vi "Main.vi"(11 "Module Admin":refnum<class "Delacor_lib_QMH_Module Admin.lvclass">) -> ()   [LabVIEW 2021, in "Hardware Selection.lvlib"]
doc: "This template is based off of the Queued Message Handler design pattern and the Queued Message Handler project template that ships with LabVIEW.\n\nThe main difference is that the queue is private to this module and communication between modules is performed via Broadcast and Request events.\n\nRequest events are wrapped in public API methods and are handled in the Event Handling Loop (EHL) of this VI. Any module can register for Broadcast events sent by this module. The EHL generates messages based on user interface actions.\n\nThe Message Handling Loop (MHL) processes messages generated by the EHL, or by other messages. The messages are string values, so new messages can be added easily to the Message Cases case structure in the MHL. Each message cluster can also provide an optional value for Message Data, which is a variant that can be converted to whatever message-specific data is required.\n_____\nBased on DQMH Project Template 7.0.1.1316."
uses:
  Hardware Selection.lvlib
  <vilib>/Delacor/Delacor QMH/Libraries/Module Admin_class/Delacor_lib_QMH_Module Admin.lvclass
  Module Data--cluster.ctl
  <vilib>/Delacor/Delacor QMH/Libraries/Message Queue_class/Delacor_lib_QMH_Message Queue.lvclass/Delacor_lib_QMH_Message Queue.ctl
  Stop Argument--cluster.ctl
  <vilib>/Delacor/Delacor QMH/Libraries/Module Admin_class/Delacor_lib_QMH_Module Admin.lvclass/Delacor_lib_QMH_Module Admin.ctl
  Get Selected RT Hardware Argument--cluster.ctl
  <vilib>/Utility/miscctls.llb/LVPointTypeDef.ctl
  Host-Control's/Module ID Action Enum.ctl
  Host-Control's/RT Exec FGV Action.ctl
  Host-Control's/DTT File's Name.ctl
  <vilib>/Delacor/Delacor QMH/Libraries/Message Queue_class/Delacor_lib_QMH_Enqueue Message (Single).vi
  <vilib>/Delacor/Delacor QMH/Libraries/Module Admin_class/Delacor_lib_QMH_Get External Launch.vi
  <userlib>/_OpenG.lib/array/array.llb/Search 1D Array (Boolean)__ogtk.vi
  <userlib>/_OpenG.lib/array/array.llb/Index 1D Array Elements (String)__ogtk.vi
  <vilib>/Delacor/Delacor QMH/Libraries/Message Queue_class/Delacor_lib_QMH_Message Queue.lvclass
  <userlib>/_OpenG.lib/array/array.llb/openg_array.lvlib
  <userlib>/_OpenG.lib/appcontrol/appcontrol.llb/openg_application_control.lvlib
panel:
  in  "DAQ-HW Selection":cluster{"Safety":bool, "Release":bool}
  in  "cDAQ-HW Data":cluster{"Hw Name":string, "Hw Ip":string}[](array[cluster])
  in  "RT-HW Selection":T1
  in  "RT-HW Data":cluster{"Hw Name":string, "Hw Ip":string}[](array[cluster])
  in  "Next":bool
  in  "Save IP":bool
  in  "Edit Tool":bool
  out "error out":errorcluster
  out "Status":string
  in  "Simulate MHL Error":bool
  in  "Simulate EHL Error":bool
  # "Hardware"
  # "IP-Address"
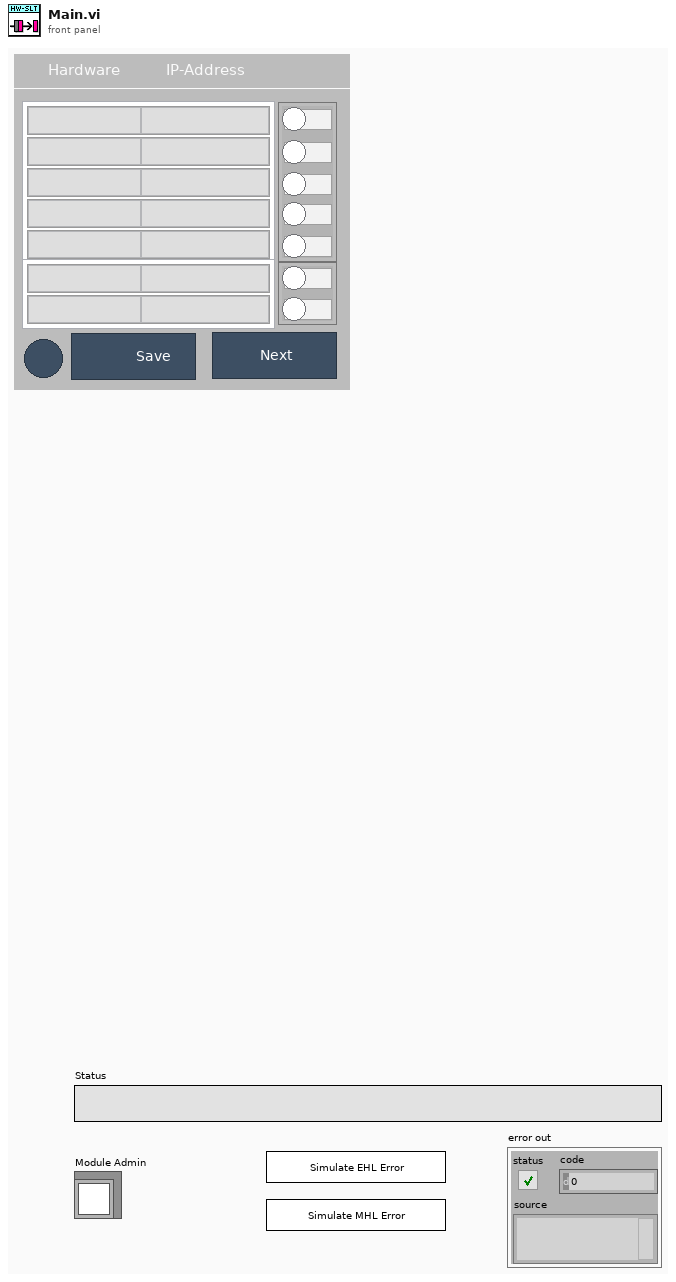
[diagram p1: front panel]
types:
  T1 = cluster{"Capsule-1":bool, "Capsule-2":bool, "Capsule-3":bool, "Capsule-4":bool, "sb-RIO":bool}
  T2 = typedef "Hardware Selection.lvlib/Request Events--cluster.ctl" = cluster{"Stop Module":refnum<user-event>, "Show Panel":refnum<user-event>, "Hide Panel":refnum<user-event>, "Get Module Execution Status":refnum<user-event>, "Show Diagram":refnum<user-event>, "Get Selected RT Hardware":refnum<user-event>}
  T3 = typedef "Hardware Selection.lvlib/Module Data--cluster.ctl" = cluster{"Status":string, "GUI Ref":cluster{"Hardware's":refnum<vi>, "IP Address":refnum<vi>}, "IP File Path":path, "HW Selection":cluster{"RT-HW Selection":cluster{"Capsule-1":bool, "Capsule-2":bool, "Capsule-3":bool, "Capsule-4":bool, "sb-RIO":bool}, "C-DAQ Hw Selection":cluster{"Safety":bool, "Release":bool}}, "IP File Data":cluster{"RT-Hw Name":string[], "cDAQ-Hw Name":string[], "RT-HW Enable?":bool[], "cDAQ-HW Enable?":bool[], "RT-HW IP":string[], "cDAQ-HW IP":string[]}, "Selected HW":cluster{"Slctd RT-Hw Name":string[], "Slctd RT-HW IP":string[], "Slctd cDAQ-Hw Name":string[], "Slctd cDAQ-HW IP":string[]}}
  T4 = cluster{"Ctrl.Label":string, "Ctrl.New Val":bool}
  T5 = enum32{"invalid lock state", "Not Locked", "Locked (No Password)", "Password-protected"}
  T6 = typedef "Hardware Selection.lvlib/Stop Argument--cluster.ctl" = cluster{"Origin":string, "Exit via Stop Module Req?":bool, "Wait for Module to stop?":bool}
  T7 = typedef "Hardware Selection.lvlib/Get Selected RT Hardware Argument--cluster.ctl" = cluster{"Get Slctd HW":bool}
  T8 = typedef "LVPointTypeDef.ctl" = cluster{"Horizontal":i16, "Vertical":i16}
  T9 = enum32{"Invalid", "Standard", "Closed", "Hidden", "Minimized", "Maximized"}
  T10 = typedef "RT Exec FGV Action.ctl" = enum16{"Init", "Insert", "Get a Exec?", "Get All Exec?"}
  T11 = typedef "Module ID Action Enum.ctl" = enum16{"Init", "Insert", "Get a ID", "Get all ID"}
  T12 = typedef "DTT File's Name.ctl" = enum16{"IP Address"}
  T13 = cluster{"RT-HW Enable?[0]":bool, "RT-HW Enable?[1]":bool, "RT-HW Enable?[2]":bool, "RT-HW Enable?[3]":bool, "RT-HW Enable?[4]":bool}
  T14 = cluster{"cDAQ-HW Enable?[0]":bool, "cDAQ-HW Enable?[1]":bool}
  T15 = cluster{"RT-Hw Name":string[], "cDAQ-Hw Name":string[], "RT-HW Enable?":bool[], "cDAQ-HW Enable?":bool[], "RT-HW IP":string[], "cDAQ-HW IP":string[]}
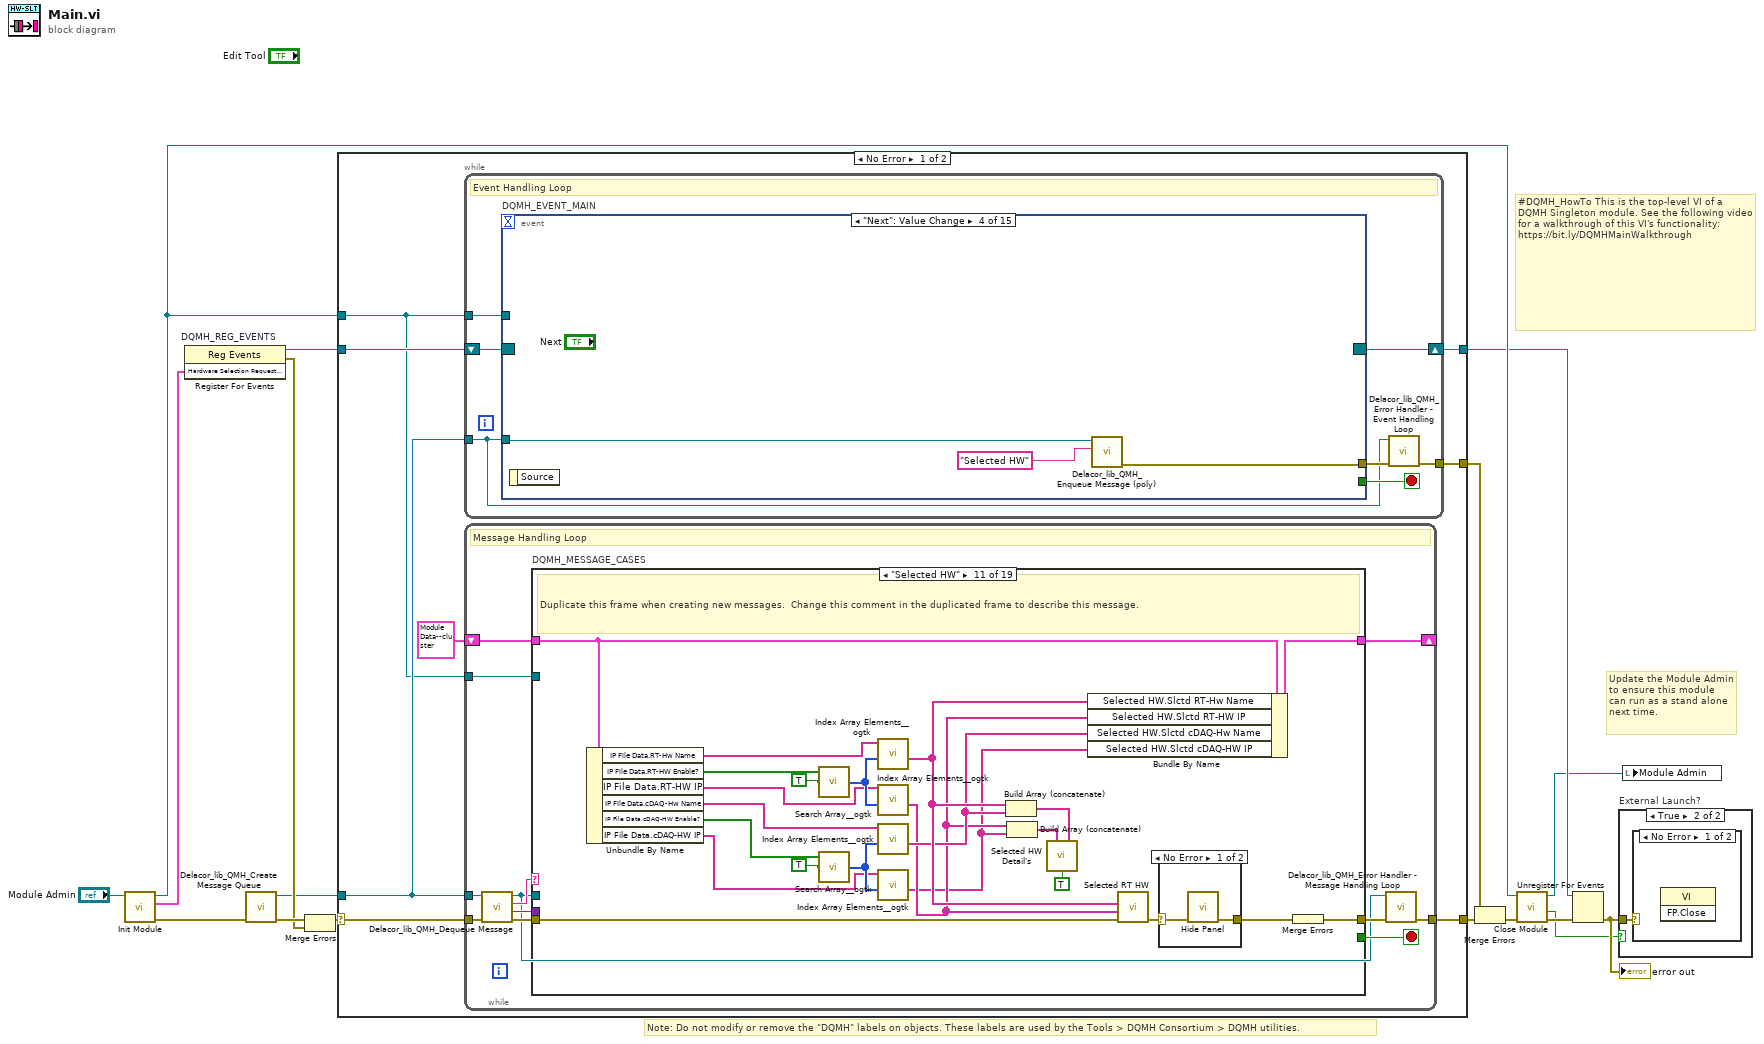
[diagram p0: block diagram]
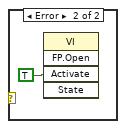
[diagram p3: hidden frame]
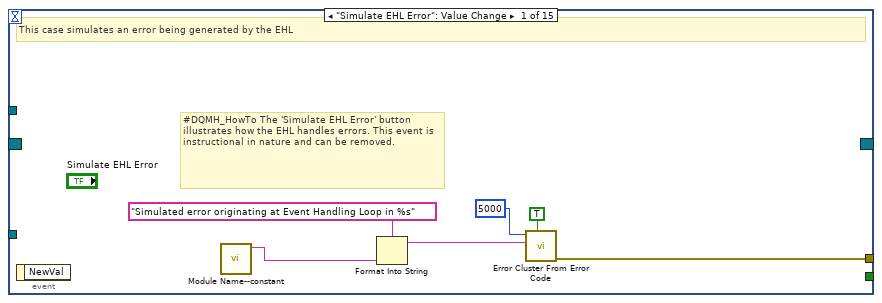
[diagram p4: hidden frame]
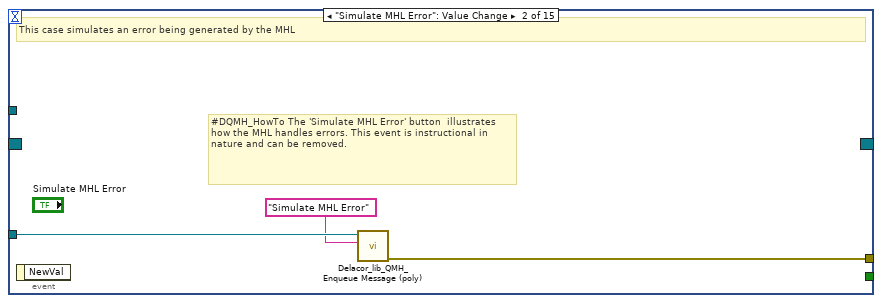
[diagram p5: hidden frame]
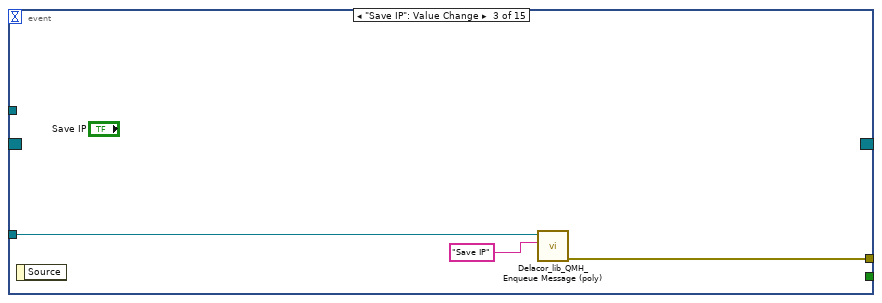
[diagram p6: hidden frame]
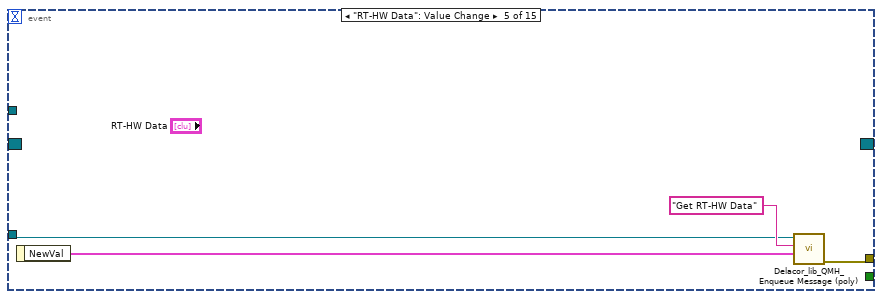
[diagram p7: hidden frame]
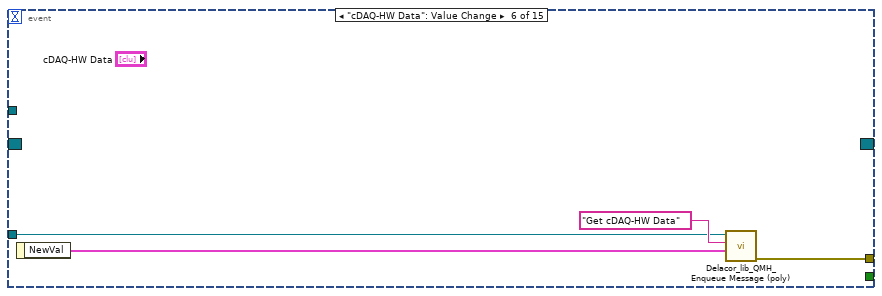
[diagram p8: hidden frame]
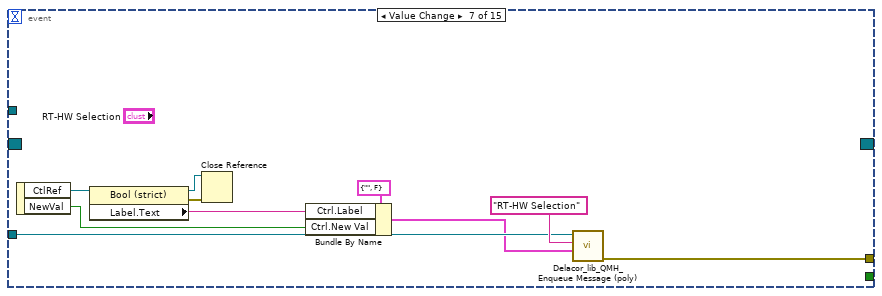
[diagram p9: hidden frame]
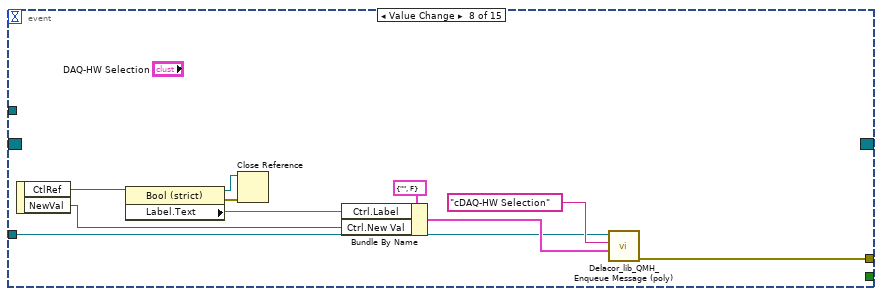
[diagram p10: hidden frame]
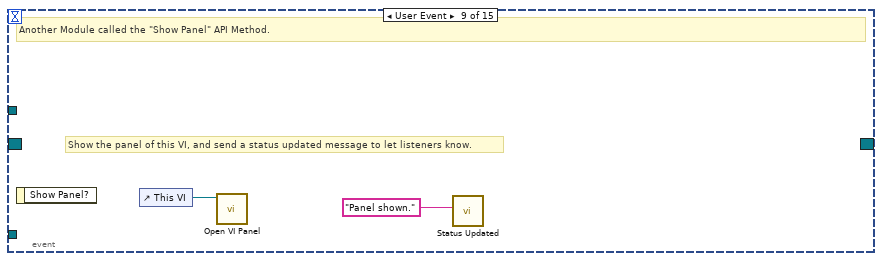
[diagram p11: hidden frame]
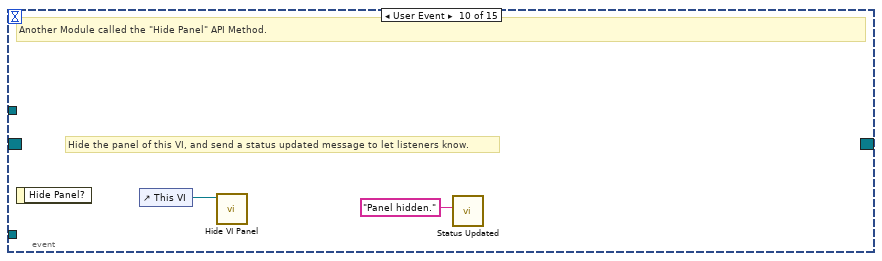
[diagram p12: hidden frame]
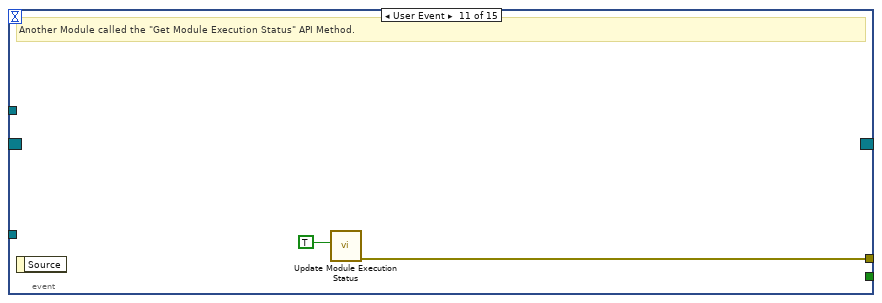
[diagram p13: hidden frame]
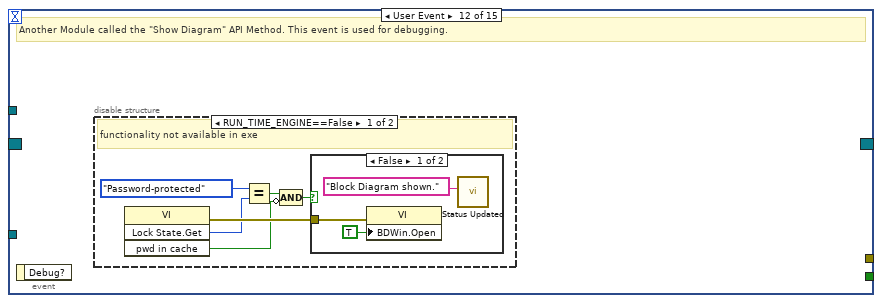
[diagram p14: hidden frame]
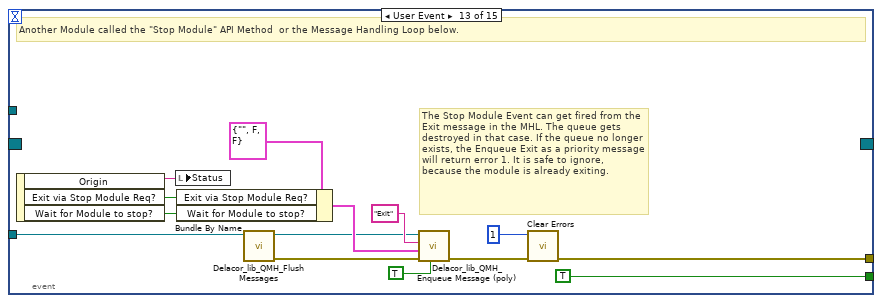
[diagram p17: hidden frame]
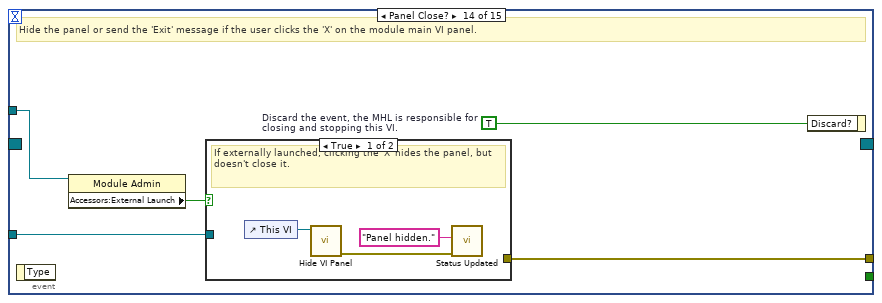
[diagram p18: hidden frame]
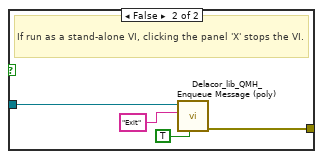
[diagram p19: hidden frame]
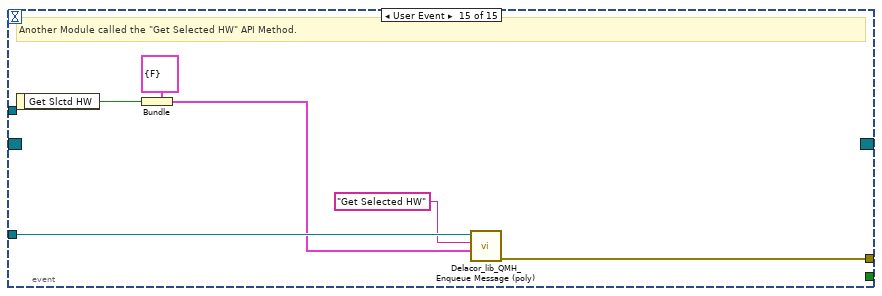
[diagram p20: hidden frame]
diagram:
  # "#DQMH_HowTo This is the top-level VI of a DQMH Singleton module. See the following video for a walkthrough of this VI's functionality: https://bit.ly/DQMHMainWalkthrough"
  # "Note: Do not modify or remove the \"DQMH\" labels on objects. These labels are used by the Tools > DQMH Consortium > DQMH utilities."
  # "Update the Module Admin to ensure this module can run as a stand alone next time."
  n1 = call "Init Module.vi"("Singleton Module Admin in"="Module Admin") -> ("error out"=w16:errorcluster, "Hardware Selection Request Events"=w5:T2, "Singleton Module Admin out"=w8:refnum<class "Delacor_lib_QMH_Module Admin.lvclass">)  [unwired: 8 in]
  n2 = register-events "DQMH_REG_EVENTS"(w5) -> (reference out=w6:refnum<event-registration>, error out=w9:errorcluster)  [unwired: 2 in]
  n3 = call <vilib>:"Delacor_lib_QMH_Create Message Queue.vi"("error in"=w16) -> ("error out"=w11:errorcluster, "Message Queue"=w4:refnum<class "Delacor_lib_QMH_Message Queue.lvclass">)  [unwired: 9 in]
  n4 = Merge Errors(w11, w9) -> (w10:errorcluster)
  n5 = case shown="No Error" w10 {
    selector: w10 -> [w23 w436]
    tunnel: [w25 w435] -> w17
    tunnel: [w22 w434] -> w7
    tunnel: w6 -> [w20 w434]
    tunnel: w4 -> [w19 w429]
    tunnel: [w24 _] -> w14
    tunnel: w8 -> [w18 w430]
    frame No Error {
      n6 = while {
        tunnel: w19 -> [w26]
        shift-right: [w29] -> w22
        shift-left: w20 -> [w30]
        tunnel: [w31] -> w24
        tunnel: w18 -> [w27]
        stop <- w28 stop-if-true
        # "Event Handling Loop"
        n7 = event "DQMH_EVENT_MAIN" shown="[3] \"Next\": Value Change" {
          selector: w30 -> [_ _ _ _ _ _ _ _ _ _ _ _ _ _ _]
          dyn-events: [_ _ _ _ _ _ _ _ _ _ _ _ _ _ _] -> w29
          timeout: _ -> [_ _ _ _ _ _ _ _ _ _ _ _ _ _ _]
          tunnel: [_ _ _ _ _ _ _ _ _ _ _ _ TRUE ("Discard?") _ _] -> w28
          tunnel: w26 -> [_ w40 w44 w45 w48 w52 w60 w66 _ _ _ _ w93 w107 w122]
          tunnel: [w38 w41 w43 w46 w50 w54 w61 w69 _ _ w81 _ w103 w109 w117] -> w32
          tunnel: w27 -> [_ _ _ _ _ _ _ _ _ _ _ _ _ w106 _]
          event "Simulate EHL Error": Value Change {
            # "#DQMH_HowTo The 'Simulate EHL Error' button  illustrates how the EHL handles errors. This event is instructional in nature and can be removed."
            # "This case simulates an error being generated by the EHL"
            n8 = event-data() -> ()  [unwired: 1 in, 1 out]
            n9 = call "Module Name--constant.vi"() -> ("Module Name"=w35:string)  [unwired: 11 in]
            n10 = Format Into String(format string="Simulated error originating at Event Handling Loop in %s", w35) -> (resulting string=w36:string)  [unwired: 2 in, 1 out]
            n11 = call <vilib>:"Error Cluster From Error Code.vi"("show call chain? (False)"=TRUE, "error message (\"\")"=w36, "error code (0)"=5000) -> ("error out"=w38:errorcluster)  [unwired: 6 in]
          }
          event "Simulate MHL Error": Value Change {
            # "#DQMH_HowTo The 'Simulate MHL Error' button  illustrates how the MHL handles errors. This event is instructional in nature and can be removed."
            # "This case simulates an error being generated by the MHL"
            n12 = event-data() -> ()  [unwired: 1 in, 1 out]
            n13 = call-poly <vilib>:"Delacor_lib_QMH_Enqueue Message (poly).vi"("Message"="Simulate MHL Error", "Message Queue in"=w40) -> ("error out"=w41:errorcluster)  [unwired: 8 in, 1 out]
          }
          event "Save IP": Value Change {
            n14 = event-data() -> ()  [unwired: 1 in, 1 out]
            n15 = call-poly <vilib>:"Delacor_lib_QMH_Enqueue Message (poly).vi"("Message"="Save IP", "Message Queue in"=w44) -> ("error out"=w43:errorcluster)  [unwired: 8 in, 1 out]
          }
          event "Next": Value Change {
            n16 = event-data() -> ()  [unwired: 1 in, 1 out]
            n17 = call-poly <vilib>:"Delacor_lib_QMH_Enqueue Message (poly).vi"("Message"="Selected HW", "Message Queue in"=w45) -> ("error out"=w46:errorcluster)  [unwired: 8 in, 1 out]
          }
          event "RT-HW Data": Value Change {
            n18 = event-data() -> ("NewVal"=w49:cluster{"Hw Name":string, "Hw Ip":string}[])  [unwired: 1 in]
            n19 = call-poly <vilib>:"Delacor_lib_QMH_Enqueue Message (poly).vi"("Message Data"=w49, "Message"="Get RT-HW Data", "Message Queue in"=w48) -> ("error out"=w50:errorcluster)  [unwired: 7 in, 1 out]
          }
          event "cDAQ-HW Data": Value Change {
            n20 = event-data() -> ("NewVal"=w53:cluster{"Hw Name":string, "Hw Ip":string}[])  [unwired: 1 in]
            n21 = call-poly <vilib>:"Delacor_lib_QMH_Enqueue Message (poly).vi"("Message Data"=w53, "Message"="Get cDAQ-HW Data", "Message Queue in"=w52) -> ("error out"=w54:errorcluster)  [unwired: 7 in, 1 out]
          }
          event "RT-HW Selection.Capsule-1", "RT-HW Selection.Capsule-2", "RT-HW Selection.Capsule-3", "RT-HW Selection.Capsule-4", "RT-HW Selection.sb-RIO": Value Change {
            n22 = event-data() -> ("CtlRef"=w65:refnum<vi>, "NewVal"=w56:bool)  [unwired: 1 in]
            n23 = property class="Bool (strict)"(reference=w65) -> (reference out=w64:refnum<vi>, error out=w63:errorcluster, "Label.Text"=w57:string)  [unwired: 1 in]
            n24 = Close Reference(reference=w64, error in (no error)=w63) -> ()  [unwired: 1 out]
            n25 = Bundle By Name(cluster=T4 {"Ctrl.Label"="", "Ctrl.New Val"=FALSE}, "Ctrl.Label"=w57, "Ctrl.New Val"=w56) -> (w58:T4)
            n26 = call-poly <vilib>:"Delacor_lib_QMH_Enqueue Message (poly).vi"("Message Data"=w58, "Message"="RT-HW Selection", "Message Queue in"=w60) -> ("error out"=w61:errorcluster)  [unwired: 7 in, 1 out]
          }
          event "DAQ-HW Selection.Safety", "DAQ-HW Selection.Release": Value Change {
            n27 = event-data() -> ("CtlRef"=w68:refnum<vi>, "NewVal"=w67:bool)  [unwired: 1 in]
            n28 = property class="Bool (strict)"(reference=w68) -> (reference out=w75:refnum<vi>, error out=w74:errorcluster, "Label.Text"=w70:string)  [unwired: 1 in]
            n29 = Close Reference(reference=w75, error in (no error)=w74) -> ()  [unwired: 1 out]
            n30 = Bundle By Name(cluster=T4 {"Ctrl.Label"="", "Ctrl.New Val"=FALSE}, "Ctrl.Label"=w70, "Ctrl.New Val"=w67) -> (w71:T4)
            n31 = call-poly <vilib>:"Delacor_lib_QMH_Enqueue Message (poly).vi"("Message Data"=w71, "Message"="cDAQ-HW Selection", "Message Queue in"=w66) -> ("error out"=w69:errorcluster)  [unwired: 7 in, 1 out]
          }
          event User Event {
            # "Show the panel of this VI, and send a status updated message to let listeners know."
            # "Another Module called the \"Show Panel\" API Method."
            n32 = event-data() -> ()  [unwired: 1 in, 1 out]
            n33 = control-ref of="This VI"() -> (w77:refnum<vi>)
            n34 = call "Open VI Panel.vi"("VI"=w77) -> ()  [unwired: 10 in, 1 out]
            n35 = call "Status Updated.vi"("Status"="Panel shown." ("format string")) -> ()  [unwired: 10 in, 1 out]
          }
          event User Event {
            # "Hide the panel of this VI, and send a status updated message to let listeners know."
            # "Another Module called the \"Hide Panel\" API Method."
            n36 = event-data() -> ()  [unwired: 1 in, 1 out]
            n37 = control-ref of="This VI"() -> (w79:refnum<vi>)
            n38 = call "Hide VI Panel.vi"("VI"=w79) -> ()  [unwired: 10 in, 1 out]
            n39 = call "Status Updated.vi"("Status"="Panel hidden." ("format string")) -> ()  [unwired: 10 in, 1 out]
          }
          event User Event {
            # "Another Module called the \"Get Module Execution Status\" API Method."
            n40 = event-data() -> ()  [unwired: 1 in, 1 out]
            n41 = call "Update Module Execution Status.vi"("Running?"=TRUE) -> ("error out"=w81:errorcluster)  [unwired: 10 in]
          }
          event User Event {
            # "Another Module called the \"Show Diagram\" API Method. This event is used for debugging."
            n42 = event-data() -> ()  [unwired: 1 in, 1 out]
            n43 = disable-structure shown="RUN_TIME_ENGINE==False" {
              frame condition #0 (active) {
                # "functionality not available in exe"
                n44 = invoke on="Invoke Node" class="VI" method="Lock State.Get"() -> (error out=w87:errorcluster, "Get Lock State"=w86:T5, "pwd in cache"=w83:bool)  [unwired: 4 in, 1 out]
                n45 = Equal?(x=T5."Password-protected", y=w86) -> (x = y?=w84:bool)
                n46 = Compound Arithmetic op=AND(w84, invert w83) -> (w82:bool)
                n47 = case shown="False" w82 {
                  tunnel: w87 -> [w90 _]
                  frame False {
                    n48 = property on="Property Node" class="VI"(error in=w90, "BDWin.Open"=TRUE ("Block Diagram Window:Open")) -> ()  [unwired: 1 in, 2 out]
                    n49 = call "Status Updated.vi"("Status"="Block Diagram shown." ("format string")) -> ()  [unwired: 10 in, 1 out]
                  }
                  frame True {
                    # "Password-protected VI, and the password is not in the cache. Do not show the diagram."
                  }
                }
              }
              frame condition #1 {
              }
            }
          }
          event User Event {
            # "The Stop Module Event can get fired from the Exit message in the MHL. The queue gets destroyed in that case. If the queue no longer exists, the Enqueue Exit as a priority message will return error 1. It is safe to ignore, because the module is already exiting."
            # "Another Module called the \"Stop Module\" API Method  or the Message Handling Loop below."
            n50 = event-data() -> ("Origin"=w100:string, "Exit via Stop Module Req?"=w96:bool, "Wait for Module to stop?"=w95:bool)  [unwired: 1 in]
            n51 = local write "Status"(w100) -> ()
            n52 = Bundle By Name(cluster=T6 {"Origin"="", "Exit via Stop Module Req?"=FALSE, "Wait for Module to stop?"=FALSE} ("Stop Argument"), "Exit via Stop Module Req?"=w96, "Wait for Module to stop?"=w95) -> (w94:T6)
            n53 = call-dynamic "Delacor_lib_QMH_Flush Messages.vi"("Message Queue in"=w93) -> ("error out"=w91:errorcluster, "Message Queue out"=w92:refnum<class "Delacor_lib_QMH_Message Queue.lvclass">)  [unwired: 7 in, 2 out]
            n54 = call-poly <vilib>:"Delacor_lib_QMH_Enqueue Message (poly).vi"("Priority Message? (F)"=TRUE, "error in"=w91, "Message Data"=w94, "Message"="Exit", "Message Queue in"=w92) -> ("error out"=w104:errorcluster)  [unwired: 5 in, 1 out]
            n55 = call <vilib>:"Clear Errors.vi"("error in (no error)"=w104, "specific error code to clear (0: all)"=1) -> ("error out"=w103:errorcluster)  [unwired: 4 in, 1 out]
          }
          event Panel Close? {
            w108 = TRUE  # Discard the event, the MHL is responsible for closing and stopping this VI.
            # "Hide the panel or send the 'Exit' message if the user clicks the 'X' on the module main VI panel."
            n56 = event-data() -> ()  [unwired: 1 in, 1 out]
            n57 = property on="Property Node" class="Module Admin"(reference=w106) -> ("Accessors:External Launch"=w105:bool)  [unwired: 1 in, 2 out]
            n58 = case shown="True" w105 {
              tunnel: w107 -> [_ w115]
              tunnel: [_ w116] -> w109
              frame True {
                # "If externally launched, clicking the 'X' hides the panel, but doesn't close it."
                n59 = control-ref of="This VI"() -> (w112:refnum<vi>)
                n60 = call "Hide VI Panel.vi"("VI"=w112) -> ("error out"=w110:errorcluster)  [unwired: 10 in]
                n61 = call "Status Updated.vi"("error in"=w110, "Status"="Panel hidden." ("format string")) -> ()  [unwired: 9 in, 1 out]
              }
              frame False {
                # "If run as a stand-alone VI, clicking the panel 'X' stops the VI."
                n62 = call-poly <vilib>:"Delacor_lib_QMH_Enqueue Message (poly).vi"("Priority Message? (F)"=TRUE, "Message"="Exit", "Message Queue in"=w115) -> ("error out"=w116:errorcluster)  [unwired: 7 in, 1 out]
              }
            }
            n63 = event-data ("Event Filter Node")("Discard?"=w108) -> ()  [unwired: 1 in, 1 out]
          }
          event User Event {
            # "Another Module called the \"Get Selected HW\" API Method."
            n64 = event-data() -> ("Get Slctd HW"=w118:bool)  [unwired: 1 in]
            n65 = Bundle(cluster=T7 {"Get Slctd HW"=FALSE} ("Get Selected HW Argument"), "Get Slctd HW"=w118) -> (w119:T7)
            n66 = call-poly <vilib>:"Delacor_lib_QMH_Enqueue Message (poly).vi"("Message Data"=w119, "Message"="Get Selected HW", "Message Queue in"=w122) -> ("error out"=w117:errorcluster)  [unwired: 7 in, 1 out]
          }
        }
        n67 = call-dynamic "Delacor_lib_QMH_Error Handler - Event Handling Loop.vi"("error in"=w32, "Message Queue in"=w26) -> ("dup error in"=w31:errorcluster)  [unwired: 8 in, 1 out]
      }
      n68 = while {
        tunnel: w19 -> [w123]
        shift-right: [w131] -> _
        shift-left: T3 {"Status"="", "GUI Ref"={"Hardware's"=refnum, "IP Address"=refnum}, "IP File Path"=path "", "HW Selection"={"RT-HW Selection"={"Capsule-1"=FALSE, "Capsule-2"=FALSE, "Capsule-3"=FALSE, "Capsule-4"=FALSE, "sb-RIO"=FALSE}, "C-DAQ Hw Selection"={"Safety"=FALSE, "Release"=FALSE}}, "IP File Data"={"RT-Hw Name"=[], "cDAQ-Hw Name"=[], "RT-HW Enable?"=[], "cDAQ-HW Enable?"=[], "RT-HW IP"=[], "cDAQ-HW IP"=[]}, "Selected HW"={"Slctd RT-Hw Name"=[], "Slctd RT-HW IP"=[], "Slctd cDAQ-Hw Name"=[], "Slctd cDAQ-HW IP"=[]}} ("Data Cluster") -> [w132]
        tunnel: w23 -> [w134]
        tunnel: [w126] -> w25
        tunnel: w18 -> [w127]
        stop <- w130 stop-if-true
        # "Message Handling Loop"
        n69 = call-dynamic "Delacor_lib_QMH_Dequeue Message.vi"("error in"=w134, "Message Queue in"=w123) -> ("error out"=w133:errorcluster, "Message Data"=w128:variant, "Message"=w129:string, "Message Queue out"=w124:refnum<class "Delacor_lib_QMH_Message Queue.lvclass">)  [unwired: 6 in]
        n70 = case "DQMH_MESSAGE_CASES" shown="\"Selected HW\"" w129 {
          selector: w129 -> [_ _ _ _ _ _ _ _ _ _ _ _ _ _ _ _ _ _ w424]
          tunnel: w124 -> [w138 w168 w182 _ _ _ _ _ _ _ _ _ w358 _ _ _ w390 w412 _]
          tunnel: w133 -> [w158 w170 w180 w194 w203 w206 w215 w230 w249 w290 w319 w341 w365 w373 w377 w386 w397 w418 w427]
          tunnel: [w139 w173 w186 w194 w195 w205 w217 w232 w251 w292 w325 w340 w368 w375 w377 w385 w393 w413 w428] -> w125
          tunnel: w132 -> [w148 w172 w185 w193 w199 w204 w213 w228 w241 w284 w316 w339 w363 w371 w376 w383 w392 w411 w425]
          tunnel: [w147 w172 w184 w193 w199 w204 w212 w227 w238 w278 w315 w339 w362 w371 w376 w383 w392 w411 w425] -> w131
          tunnel: [_ _ _ _ _ _ _ _ _ _ _ _ _ _ _ _ _ w410 _] -> w130
          tunnel: w128 -> [_ _ _ _ w202 _ w216 w231 w250 w291 _ _ _ _ _ _ w391 w409 _]
          tunnel: w127 -> [w149 _ _ _ _ _ _ _ _ _ _ _ _ _ _ _ w389 w404 _]
          frame "Initialize" {
            w143 = "Initial Message" ("Initial Message")
            # "#CodeNeeded - Initialize the appearance of the front panel."
            # "#CodeNeeded - Initialize your state data here."
            # "Initialize - Any operation that needs to be done before the module can receive messages. Synchronize Caller Events.vi will inform Start Module.vi that the module has launched and is ready to receive messages. Module Did Init.vi will broadcast that the module initialized."
            n71 = call "Synchronize Caller Events.vi"("error in"=w158, "Singleton Module Admin in"=w149) -> ("error out"=w157:errorcluster, "Singleton Module Admin out"=w144:refnum<class "Delacor_lib_QMH_Module Admin.lvclass">)  [unwired: 8 in]
            n72 = property on="Property Node" class="Module Admin"(reference=w144) -> ("Accessors:External Launch"=w153:bool)  [unwired: 1 in, 2 out]
            n73 = Select(t=T9."Hidden" ("State"), s=w153, f=T9."Standard" ("State")) -> (s? t:f=w150:T9)
            n74 = control-ref of="This VI"() -> (w137:refnum<vi>)
            n75 = call "Module Name--constant.vi"() -> ("Module Name"=w156:string)  [unwired: 11 in]
            n76 = property on="Property Node" class="VI"(reference=w137, "Front Panel.Title"=w156) -> (reference out=w155:refnum<vi>, error out=w160:errorcluster)  [unwired: 1 in]
            n77 = call "Module Name--constant.vi"() -> ("Module Name"=w145:string)  [unwired: 11 in]
            n78 = invoke on="Invoke Node" class="VI" method="FP.Open"(reference=w155, error in=w160, "State"=w150) -> (reference out=w154:refnum<vi>, error out=w159:errorcluster)  [unwired: 2 in, 3 out]
            n79 = Bundle By Name(cluster=w148, "Status"=w143) -> (w147:T3)
            n80 = call "Module Did Init.vi"("error in"=w157, "Initialized?"=TRUE, "Origin"=w145) -> ("error out"=w140:errorcluster)  [unwired: 8 in]
            n81 = invoke on="Invoke Node" class="VI" method="FP.Center"(reference=w154, error in=w159) -> ()  [unwired: 1 in, 3 out]
            n82 = property on="Pane" class="Pane"("Origin"=T8 {"Horizontal"=0, "Vertical"=0}) -> (error out=w136:errorcluster)  [unwired: 2 in, 1 out]
            n83 = call-poly <vilib>:"Delacor_lib_QMH_Enqueue Message (poly).vi"("error in"=w140, "Message"="Init-1", "Message Queue in"=w138) -> ("error out"=w139:errorcluster)  [unwired: 7 in, 1 out]
            n84 = call <userlib>:"Fit VI window to Largest Dec__ogtk.vi"("error in (no error)"=w136) -> ("error out"=w135:errorcluster)  [unwired: 5 in, 1 out]
            n85 = call <vilib>:"Clear Errors.vi"("error in (no error)"=w135) -> ()  [unwired: 5 in, 2 out]
            "Status" <- w143
          }
          frame "Init-1" {
            # "Duplicate this frame when creating new messages.  Change this comment in the duplicated frame to describe this message."
            n86 = call "Folder Creation.vi"("Create New? (F)"=TRUE) -> ("error out"=w166:errorcluster)  [unwired: 12 in, 2 out]
            n87 = call "File Path's.vi"("Create New? (F)"=TRUE, "error in"=w166) -> ("error out"=w163:errorcluster)  [unwired: 12 in, 1 out]
            n88 = call "RT Execution State.vi"("error in"=w163, "Action"=RT_Exec_FGV_Action."Init") -> ("error out"=w162:errorcluster)  [unwired: 10 in, 3 out]
            n89 = call "RT Module ID.vi"("error in"=w162, "Action"=Module_ID_Action_Enum."Init") -> ()  [unwired: 10 in, 4 out]
            n90 = call-poly <vilib>:"Delacor_lib_QMH_Enqueue Message (poly).vi"("error in"=w170, "Message"="Init-2", "Message Queue in"=w168) -> ("error out"=w169:errorcluster)  [unwired: 7 in, 1 out]
            n91 = Merge Errors(w169) -> (w173:errorcluster)
          }
          frame "Init-2" {
            w174 = string[] ["Safety", "Release"] ("Hw Name")
            w176 = string[] ["Capsule-1", "Capsule-2", "Capsule-3", "Capsule-4", "sb-RIO"] ("Hw Name")
            # "Duplicate this frame when creating new messages.  Change this comment in the duplicated frame to describe this message."
            n92 = for {
              tunnel: w176 -> [w192] mode=indexing
              tunnel: [w191] -> w177 mode=indexing
              n93 = Bundle("Hw Name"=w192, "HW IP"="") -> (w191:cluster{"Hw Name":string, "HW IP":string})  [unwired: 1 in]
            }
            n94 = for {
              tunnel: w174 -> [w189] mode=indexing
              tunnel: [w188] -> w175 mode=indexing
              n95 = Bundle("Hw Name"=w189, "HW IP"="") -> (w188:cluster{"Hw Name":string, "HW IP":string})  [unwired: 1 in]
            }
            n96 = property on="RT-HW Data" class="Arr (strict)"("Value"=w177) -> ()  [unwired: 2 in, 2 out]
            n97 = property on="cDAQ-HW Data" class="Arr (strict)"("Value"=w175) -> ()  [unwired: 2 in, 2 out]
            n98 = call "File Path's.vi"("File Name"=DTT_File's_Name."IP Address") -> ("File Path Out"=w178:path)  [unwired: 13 in, 1 out]
            n99 = call-poly <vilib>:"Delacor_lib_QMH_Enqueue Message (poly).vi"("error in"=w180, "Message"="Read IP File", "Message Queue in"=w182) -> ("error out"=w181:errorcluster)  [unwired: 7 in, 1 out]
            n100 = Bundle By Name(cluster=w185, "IP File Data.RT-Hw Name"=w176, "IP File Path"=w178, "IP File Data.cDAQ-Hw Name"=w174) -> (w184:T3)
            n101 = Merge Errors(w181) -> (w186:errorcluster)
          }
          frame "---Module Specific---" {
            # "Separator -- The following cases handle messages specific to this Module."
          }
          frame "Get Selected HW" {
            # "This Request event will request the Hardware Selection Module to send the Selected Hardware to all the module's which need this list."
            n102 = Variant To Data(error in=w203, type=T7 {"Get Slctd HW"=FALSE} ("Get Selected HW Argument"), Variant=w202) -> (data=w200:T7, error out=w196:errorcluster)
            n103 = Unbundle By Name(w200) -> ()  [unwired: 1 out]
            n104 = Unbundle By Name(w199) -> ("Selected HW.Slctd RT-Hw Name"=w198:string[], "Selected HW.Slctd RT-HW IP"=w197:string[])
            n105 = call "Selected RT HW.vi"("error in"=w196, "Slctd HW IP"=w197, "Slctd Hw Name"=w198) -> ("error out"=w195:errorcluster)  [unwired: 8 in]
          }
          frame "---Copy This Frame---" {
            # "Duplicate this frame when creating new messages.  Change this comment in the duplicated frame to describe this message."
            n106 = Merge Errors(w206) -> (w205:errorcluster)
          }
          frame "Get RT-HW Data" {
            # "Duplicate this frame when creating new messages.  Change this comment in the duplicated frame to describe this message."
            n107 = Variant To Data(error in=w215, type=cluster{"Hw Name":string, "Hw Ip":string}[] [] ("NewVal"), Variant=w216) -> (data=w211:cluster{"Hw Name":string, "Hw Ip":string}[], error out=w209:errorcluster)
            n108 = for {
              tunnel: w211 -> [w221] mode=indexing
              tunnel: [w220] -> w208 mode=indexing
              tunnel: [w219] -> w207 mode=indexing
              shift-right: [w218] -> w210
              shift-left: w209 -> [w218]
              n109 = Unbundle By Name(w221) -> ("Hw Name"=w220:string, "Hw Ip"=w219:string)
            }
            n110 = Bundle By Name(cluster=w213, "IP File Data.RT-Hw Name"=w208, "IP File Data.RT-HW IP"=w207) -> (w212:T3)
            n111 = Merge Errors(w210) -> (w217:errorcluster)
          }
          frame "Get cDAQ-HW Data" {
            # "Duplicate this frame when creating new messages.  Change this comment in the duplicated frame to describe this message."
            n112 = Variant To Data(error in=w230, type=cluster{"Hw Name":string, "Hw Ip":string}[] [] ("NewVal"), Variant=w231) -> (data=w226:cluster{"Hw Name":string, "Hw Ip":string}[], error out=w224:errorcluster)
            n113 = for {
              tunnel: w226 -> [w236] mode=indexing
              tunnel: [w235] -> w223 mode=indexing
              tunnel: [w234] -> w222 mode=indexing
              shift-right: [w233] -> w225
              shift-left: w224 -> [w233]
              n114 = Unbundle By Name(w236) -> ("Hw Name"=w235:string, "Hw Ip"=w234:string)
            }
            n115 = Bundle By Name(cluster=w228, "IP File Data.cDAQ-Hw Name"=w223, "IP File Data.cDAQ-HW IP"=w222) -> (w227:T3)
            n116 = Merge Errors(w225) -> (w232:errorcluster)
          }
          frame "RT-HW Selection" {
            # "Duplicate this frame when creating new messages.  Change this comment in the duplicated frame to describe this message."
            n117 = Variant To Data(error in=w249, type=T4 {"Ctrl.Label"="", "Ctrl.New Val"=FALSE}, Variant=w250) -> (data=w247:T4, error out=w246:errorcluster)
            n118 = Unbundle By Name(w247) -> ("Ctrl.Label"=w243:string, "Ctrl.New Val"=w242:bool)
            n119 = case shown="\"Capsule-3\"" w243 {
              tunnel: w246 -> [w252 w258 w263 w268 w273 w277]
              tunnel: [w252 w258 w263 w268 w273 w277] -> w245
              tunnel: w242 -> [_ w255 w260 w265 w270 w274]
              tunnel: w241 -> [w253 w257 w262 w267 w272 w276]
              tunnel: [w253 w256 w261 w266 w271 w275] -> w239
              frame Default {
              }
              frame "Capsule-1" {
                w254 = FALSE ("HW Selection.RT-HW Selection.Capsule-2")
                n120 = Bundle By Name(cluster=w257, "HW Selection.RT-HW Selection.Capsule-2"=w254, "HW Selection.RT-HW Selection.Capsule-3"=w254, "HW Selection.RT-HW Selection.Capsule-4"=w254, "HW Selection.RT-HW Selection.Capsule-1"=w255) -> (w256:T3)
              }
              frame "Capsule-2" {
                w259 = FALSE ("HW Selection.RT-HW Selection.Capsule-2")
                n121 = Bundle By Name(cluster=w262, "HW Selection.RT-HW Selection.Capsule-1"=w259, "HW Selection.RT-HW Selection.Capsule-3"=w259, "HW Selection.RT-HW Selection.Capsule-4"=w259, "HW Selection.RT-HW Selection.Capsule-2"=w260) -> (w261:T3)
              }
              frame "Capsule-3" {
                w264 = FALSE ("HW Selection.RT-HW Selection.Capsule-2")
                n122 = Bundle By Name(cluster=w267, "HW Selection.RT-HW Selection.Capsule-1"=w264, "HW Selection.RT-HW Selection.Capsule-2"=w264, "HW Selection.RT-HW Selection.Capsule-4"=w264, "HW Selection.RT-HW Selection.Capsule-3"=w265) -> (w266:T3)
              }
              frame "Capsule-4" {
                w269 = FALSE ("HW Selection.RT-HW Selection.Capsule-2")
                n123 = Bundle By Name(cluster=w272, "HW Selection.RT-HW Selection.Capsule-1"=w269, "HW Selection.RT-HW Selection.Capsule-2"=w269, "HW Selection.RT-HW Selection.Capsule-3"=w269, "HW Selection.RT-HW Selection.Capsule-4"=w270) -> (w271:T3)
              }
              frame "sb-RIO" {
                n124 = Bundle By Name(cluster=w276, "HW Selection.RT-HW Selection.sb-RIO"=w274) -> (w275:T3)
              }
            }
            n125 = Unbundle By Name(w239) -> ("HW Selection.RT-HW Selection"=w240:T1)
            n126 = Cluster To Array(cluster=w240) -> (array=w237:bool[])
            n127 = Bundle By Name(cluster=w239, "IP File Data.RT-HW Enable?"=w237) -> (w238:T3)
            n128 = property on="RT-HW Selection" class="Clust (strict)"(error in=w245, "Value"=w240) -> (error out=w244:errorcluster)  [unwired: 1 in, 1 out]
            n129 = Merge Errors(w244) -> (w251:errorcluster)
          }
          frame "cDAQ-HW Selection" {
            # "Duplicate this frame when creating new messages.  Change this comment in the duplicated frame to describe this message."
            n130 = Variant To Data(error in=w290, type=T4 {"Ctrl.Label"="", "Ctrl.New Val"=FALSE}, Variant=w291) -> (data=w288:T4, error out=w287:errorcluster)
            n131 = Unbundle By Name(w288) -> ("Ctrl.Label"=w286:string, "Ctrl.New Val"=w285:bool)
            n132 = case shown="\"Release\"" w286 {
              tunnel: w287 -> [w293 w298 w302]
              tunnel: [w293 w298 w302] -> w283
              tunnel: w285 -> [_ w295 w299]
              tunnel: w284 -> [w294 w297 w301]
              tunnel: [w294 w296 w300] -> w280
              frame Default {
              }
              frame "Safety" {
                n133 = Bundle By Name(cluster=w297, "HW Selection.C-DAQ Hw Selection.Safety"=w295) -> (w296:T3)
              }
              frame "Release" {
                n134 = Bundle By Name(cluster=w301, "HW Selection.C-DAQ Hw Selection.Release"=w299) -> (w300:T3)
              }
            }
            n135 = Unbundle By Name(w280) -> ("HW Selection.C-DAQ Hw Selection"=w281:cluster{"Safety":bool, "Release":bool})
            n136 = Cluster To Array(cluster=w281) -> (array=w279:bool[])
            n137 = Bundle By Name(cluster=w280, "IP File Data.cDAQ-HW Enable?"=w279) -> (w278:T3)
            n138 = property on="DAQ-HW Selection" class="Clust (strict)"(error in=w283, "Value"=w281) -> (error out=w282:errorcluster)  [unwired: 1 in, 1 out]
            n139 = Merge Errors(w282) -> (w292:errorcluster)
          }
          frame "Selected HW" {
            # "Duplicate this frame when creating new messages.  Change this comment in the duplicated frame to describe this message."
            n140 = Unbundle By Name(w316) -> ("IP File Data.RT-Hw Name"=w321:string[], "IP File Data.RT-HW Enable?"=w324:bool[], "IP File Data.RT-HW IP"=w320:string[], "IP File Data.cDAQ-Hw Name"=w312:string[], "IP File Data.cDAQ-HW Enable?"=w311:bool[], "IP File Data.cDAQ-HW IP"=w310:string[])
            n141 = call-poly <userlib>:"Search Array__ogtk.vi"("Array"=w324, "Element Data"=TRUE) -> ("Indices of Elements"=w322:i32[])  [unwired: 7 in]
            n142 = call-poly <userlib>:"Search Array__ogtk.vi"("Array"=w311, "Element Data"=TRUE) -> ("Indices of Elements"=w314:i32[])  [unwired: 7 in]
            n143 = call-poly <userlib>:"Index Array Elements__ogtk.vi"("indices"=w322, "array"=w321) -> ("elements"=w309:string[])  [unwired: 9 in]
            n144 = call-poly <userlib>:"Index Array Elements__ogtk.vi"("indices"=w322, "array"=w320) -> ("elements"=w306:string[])  [unwired: 9 in]
            n145 = call-poly <userlib>:"Index Array Elements__ogtk.vi"("indices"=w314, "array"=w312) -> ("elements"=w308:string[])  [unwired: 9 in]
            n146 = call-poly <userlib>:"Index Array Elements__ogtk.vi"("indices"=w314, "array"=w310) -> ("elements"=w305:string[])  [unwired: 9 in]
            n147 = Build Array (concatenate)(w309, w308) -> (w307:string[])
            n148 = Build Array (concatenate)(w306, w305) -> (w304:string[])
            n149 = call "Selected HW Detail's.vi"("HW IP"=w304, "HW Name"=w307, "Write(F)"=TRUE) -> ()  [unwired: 10 in, 3 out]
            n150 = Bundle By Name(cluster=w316, "Selected HW.Slctd RT-Hw Name"=w309, "Selected HW.Slctd RT-HW IP"=w306, "Selected HW.Slctd cDAQ-Hw Name"=w308, "Selected HW.Slctd cDAQ-HW IP"=w305) -> (w315:T3)
            n151 = call "Selected RT HW.vi"("error in"=w319, "Slctd HW IP"=w306, "Slctd Hw Name"=w309) -> ("error out"=w318:errorcluster)  [unwired: 8 in]
            n152 = case shown="No Error" w318 {
              selector: w318 -> [w327 w328]
              tunnel: [w326 w328] -> w317
              frame No Error {
                n153 = call "Hide Panel.vi"("error in"=w327) -> ("error out"=w326:errorcluster)  [unwired: 10 in]
              }
              frame Error {
              }
            }
            n154 = Merge Errors(w317) -> (w325:errorcluster)
          }
          frame "Update GUI" {
            # "Duplicate this frame when creating new messages.  Change this comment in the duplicated frame to describe this message."
            n155 = Unbundle By Name(w339) -> ("IP File Data.RT-HW Enable?"=w338:bool[], "IP File Data.RT-Hw Name"=w337:string[], "IP File Data.RT-HW IP"=w336:string[], "IP File Data.cDAQ-Hw Name"=w333:string[], "IP File Data.cDAQ-HW IP"=w332:string[], "IP File Data.cDAQ-HW Enable?"=w330:bool[])
            n156 = Array To Cluster(array=w338) -> (cluster=w334:T13)
            n157 = Array To Cluster(array=w330) -> (cluster=w329:T14)
            n158 = for {
              tunnel: w337 -> [w351] mode=indexing
              tunnel: w336 -> [w349]
              tunnel: [w350] -> w335 mode=indexing
              i -> [w348]
              n159 = Index Array(array=w349, index=w348) -> (element=w347:string)
              n160 = Bundle("Hw Name"=w351, "HW IP"=w347) -> (w350:cluster{"Hw Name":string, "HW IP":string})  [unwired: 1 in]
            }
            n161 = for {
              tunnel: w333 -> [w346] mode=indexing
              tunnel: w332 -> [w344]
              tunnel: [w345] -> w331 mode=indexing
              i -> [w343]
              n162 = Index Array(array=w344, index=w343) -> (element=w342:string)
              n163 = Bundle("Hw Name"=w346, "HW IP"=w342) -> (w345:cluster{"Hw Name":string, "HW IP":string})  [unwired: 1 in]
            }
            n164 = property on="RT-HW Selection" class="Clust (strict)"("Value"=w334) -> ()  [unwired: 2 in, 2 out]
            n165 = property on="DAQ-HW Selection" class="Clust (strict)"("Value"=w329) -> ()  [unwired: 2 in, 2 out]
            n166 = property on="RT-HW Data" class="Arr (strict)"("Value"=w335) -> ()  [unwired: 2 in, 2 out]
            n167 = property on="cDAQ-HW Data" class="Arr (strict)"("Value"=w331) -> ()  [unwired: 2 in, 2 out]
            n168 = Merge Errors(w341) -> (w340:errorcluster)
          }
          frame "Read IP File" {
            w357 = T15 {"RT-Hw Name"=[], "cDAQ-Hw Name"=[], "RT-HW Enable?"=[], "cDAQ-HW Enable?"=[], "RT-HW IP"=[], "cDAQ-HW IP"=[]} ("IP File Data")
            # "Duplicate this frame when creating new messages.  Change this comment in the duplicated frame to describe this message."
            n169 = Unbundle By Name(w363) -> ("IP File Path"=w364:path)
            n170 = call <vilib>:"Easy Read XML File__JKI EasyXML.vi"("error in (no error)"=w365, "LabVIEW Data (Type)"=w357, "XML File Path"=w364) -> ("error out"=w366:errorcluster, "LabVIEW Data"=w367:variant)  [unwired: 6 in, 1 out]
            n171 = Variant To Data(error in=w366, type=w357, Variant=w367) -> (data=w356:T15, error out=w360:errorcluster)
            n172 = Unbundle By Name(w356) -> ("RT-HW Enable?"=w355:bool[], "RT-HW IP"=w354:string[], "cDAQ-HW Enable?"=w353:bool[], "cDAQ-HW IP"=w352:string[])
            n173 = Bundle By Name(cluster=w363, "IP File Data.RT-HW Enable?"=w355, "IP File Data.RT-HW IP"=w354, "IP File Data.cDAQ-HW Enable?"=w353, "IP File Data.cDAQ-HW IP"=w352) -> (w362:T3)
            n174 = call-poly <vilib>:"Delacor_lib_QMH_Enqueue Message (poly).vi"("error in"=w360, "Message"="Update GUI", "Message Queue in"=w358) -> ("error out"=w359:errorcluster)  [unwired: 7 in, 1 out]
            n175 = Merge Errors(w359) -> (w368:errorcluster)
          }
          frame "Save IP" {
            # "Duplicate this frame when creating new messages.  Change this comment in the duplicated frame to describe this message."
            n176 = Unbundle By Name(w371) -> ("IP File Path"=w370:path, "IP File Data"=w369:T15)
            n177 = call <vilib>:"Easy Write XML File__JKI EasyXML.vi"("error in (no error)"=w373, "Overwrite File? (false)"=TRUE, "LabVIEW Data"=w369, "XML File Path"=w370) -> ("error out"=w374:errorcluster)  [unwired: 6 in, 1 out]
            n178 = Merge Errors(w374) -> (w375:errorcluster)
          }
          frame "---Exit and Error Handling---" {
            # "Separator - The following cases handle errors and exit messages."
          }
          frame "Simulate MHL Error" {
            # "#DQMH_HowTo The 'Simulate MHL Error' button  illustrates how the MHL handles errors. This event is instructional in nature and can be removed."
            # "Simulate an error occurring at the MHL"
            n179 = call "Module Name--constant.vi"() -> ("Module Name"=w379:string)  [unwired: 11 in]
            n180 = Format Into String(format string="Simulated error originating at Message Handling Loop in %s", w379) -> (resulting string=w380:string)  [unwired: 2 in, 1 out]
            n181 = call <vilib>:"Error Cluster From Error Code.vi"("show call chain? (False)"=TRUE, "error message (\"\")"=w380, "error code (0)"=5001) -> ("error out"=w384:errorcluster)  [unwired: 6 in]
            n182 = Merge Errors(w386, w384) -> (w385:errorcluster)
          }
          frame "Error" {
            # "#CodeRecommended - If the module is running in standalone mode (External Launch = FALSE), this code will pop up an error dialog and call the 'Exit' message if an error occurs. Add more fine-grained error management here."
            # "Error - Check the error message data and respond accordingly. This message is sent by the \"Error Handler\" VIs at the end of each loop in this application."
            n183 = Variant To Data(error in=w397, type=errorcluster {"status"=FALSE, "code"=0, "source"=""} ("error constant"), Variant=w391) -> (data=w387:errorcluster, error out=w395:errorcluster)
            n184 = property on="Property Node" class="Module Admin"(reference=w389) -> ("Accessors:External Launch"=w388:bool)  [unwired: 1 in, 2 out]
            n185 = local write "error out"(w387) -> ()
            n186 = call "Error Reported.vi"("Error"=w387) -> ()  [unwired: 10 in, 1 out]
            n187 = case shown="False" w388 {
              tunnel: [w402 _] -> w394
              tunnel: w390 -> [w400 _]
              tunnel: w387 -> [w401 _]
              frame False {
                n188 = disable-structure shown="Default" {
                  disable-tunnel: w401 -> [w403 _]
                  frame condition #0 (active) {
                    # "If the module is running standalone, then pop up an error dialog and call the \"Exit\" message."
                    n189 = call <vilib>:"Simple Error Handler.vi"("error in (no error)"=w403) -> ()  [unwired: 4 in, 5 out]
                  }
                  frame condition #1 {
                    # "To prevent the Simple Error Handler VI from being loaded (e.g. when deploying to a Real-Time target), add the Conditional Disable Symbol \"DQMH_Disable_SEH\" to your project and set it to TRUE."
                  }
                }
                n190 = call-poly <vilib>:"Delacor_lib_QMH_Enqueue Message (poly).vi"("Priority Message? (F)"=TRUE, "Message"="Exit", "Message Queue in"=w400) -> ("error out"=w402:errorcluster)  [unwired: 7 in, 1 out]
              }
              frame True {
                # "If the module was launched externally, calling the Error Reported broadcast VI is the only action performed by the \"Error\" message. The module's caller can then process the error appropriately."
              }
            }
            n191 = Merge Errors(w395, w394) -> (w393:errorcluster)
          }
          frame "Exit" {
            w408 = 91  # 91: not all Exit messages will have an argument
            w410 = TRUE  # Stop the VI
            # "Release the message queue reference"
            # "#CodeNeeded - Add any required cleanup code here."
            # "Exit - Exit the application."
            n192 = Variant To Data(error in=w418, type=T6 {"Origin"="", "Exit via Stop Module Req?"=FALSE, "Wait for Module to stop?"=FALSE} ("Stop Argument"), Variant=w409) -> (data=w406:T6, error out=w415:errorcluster)
            n193 = call <vilib>:"Clear Errors.vi"("error in (no error)"=w415, "specific error code to clear (0: all)"=w408) -> ("error out"=w417:errorcluster)  [unwired: 4 in, 1 out]
            n194 = control-ref of="This VI"() -> (w405:refnum<vi>)
            n195 = call-dynamic "Delacor_lib_QMH_Release Message Queue.vi"("error in"=w417, "Message Queue"=w412) -> ("error out"=w416:errorcluster)  [unwired: 9 in]
            n196 = call "Handle Exit.vi"("Stop Argument"=w406, "Admin in"=w404, "VI reference"=w405) -> ("error out"=w414:errorcluster)  [unwired: 7 in, 1 out]
            n197 = Merge Errors(w416, w414) -> (w413:errorcluster)
            n198 = call "Error Reported.vi"("Error"=w413) -> ()  [unwired: 10 in, 1 out]
          }
          frame Default {
            # "'Default' case only runs if there is a message that isn't defined in any of the other cases.  Output a programming error."
            n199 = call "Module Name--constant.vi"() -> ("Module Name"=w423:string)  [unwired: 11 in]
            n200 = Format Into String(format string="The invalid message string \"%s\" was received in the Message Handling Loop for module \"%s\".", w424, w423) -> (resulting string=w419:string)  [unwired: 2 in, 1 out]
            n201 = call <vilib>:"Error Cluster From Error Code.vi"("show call chain? (False)"=TRUE, "error message (\"\")"=w419, "error code (0)"=1) -> ("error out"=w426:errorcluster)  [unwired: 6 in]
            n202 = Merge Errors(w427, w426) -> (w428:errorcluster)
          }
        }
        n203 = call-dynamic "Delacor_lib_QMH_Error Handler - Message Handling Loop.vi"("error in"=w125, "Message Queue in"=w124) -> ("dup error in"=w126:errorcluster)  [unwired: 8 in, 1 out]
      }
    }
    frame Error {
      # "Synchronize Caller Events.vi will inform Start Module.vi that the module has launched and will let the code calling Start Module.vi register for broadcasts and would permit the caller receive the broadcast that an error occurred at launch time."
      n204 = call-dynamic "Delacor_lib_QMH_Release Message Queue.vi"("error in"=w436, "Message Queue"=w429) -> ("error out"=w435:errorcluster)  [unwired: 9 in]
      n205 = call "Synchronize Caller Events.vi"("Singleton Module Admin in"=w430) -> ("error out"=w437:errorcluster)  [unwired: 9 in, 1 out]
      n206 = call "Module Name--constant.vi"() -> ("Module Name"=w433:string)  [unwired: 11 in]
      n207 = Format Into String(format string="An error occurred during initialization. %s is no longer running.", w433) -> (resulting string=w431:string)  [unwired: 2 in, 1 out]
      n208 = Merge Errors(w435, w437) -> (w438:errorcluster)
      n209 = call "Error Reported.vi"("Additional Information"=w431, "Error"=w438) -> ()  [unwired: 9 in, 1 out]
    }
  }
  n210 = Merge Errors(w14, w17) -> (w13:errorcluster)
  n211 = call "Close Module.vi"("error in"=w13, "Module Admin in"=w8) -> ("error out"=w15:errorcluster, "External Launch"=w1:bool, "Module Admin out"=w2:refnum<class "Delacor_lib_QMH_Module Admin.lvclass">)  [unwired: 7 in]
  n212 = Unregister For Events(event registration refnum=w7, error in=w15) -> (error out=w12:errorcluster)
  "error out" <- w12
  n213 = case "External Launch?" shown="True" w1 {
    tunnel: w12 -> [_ w439]
    frame False {
    }
    frame True {
      n214 = case shown="No Error" w439 {
        frame No Error {
          n215 = invoke on="Invoke Node" class="VI" method="FP.Close"() -> ()  [unwired: 3 in, 3 out]
        }
        frame Error {
          n216 = invoke on="Invoke Node" class="VI" method="FP.Open"("Activate"=TRUE ("Activate?")) -> ()  [unwired: 4 in, 5 out]
        }
      }
    }
  }
  n217 = local write "Module Admin"(w2) -> ()
